vi "Write Count.vi"(8 "error in (no error)":errorcluster, 10 "Count":bool, 11 "TileTimer in":refnum<class "TileTimer.lvclass">) -> (0 "error out":errorcluster, 3 "TileTimer out":refnum<class "TileTimer.lvclass">)   [LabVIEW 2019, in "RT_Game.lvlib" / "TileTimer.lvclass"]
uses:
  TileTimer.lvclass
  TileTimer.lvclass/TileTimer.ctl
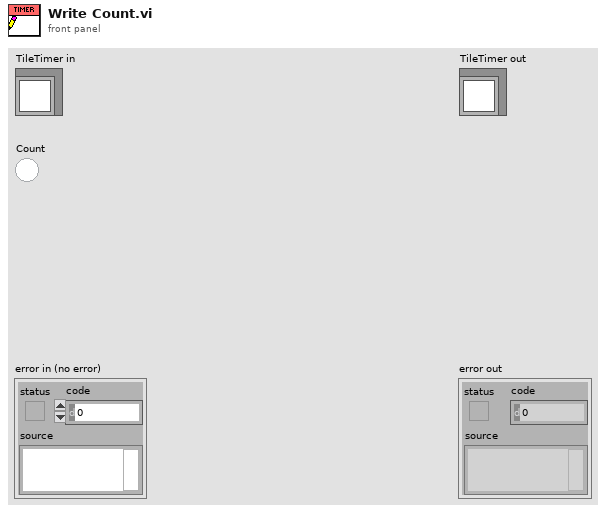
[diagram p1: front panel]
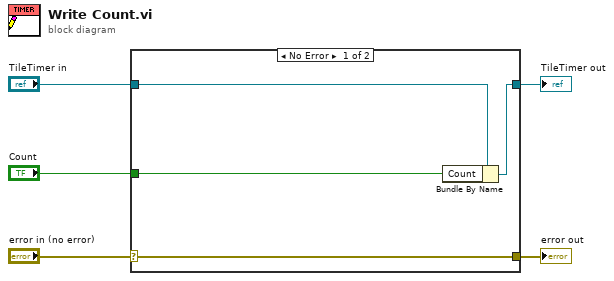
[diagram p0: block diagram]
diagram:
  n1 = case shown="No Error" "error in (no error)" {
    selector: "error in (no error)" -> [w9 w10]
    tunnel: [w9 w10] -> w4
    tunnel: [w7 w11] -> w2
    tunnel: "TileTimer in" -> [w8 w11]
    tunnel: "Count" -> [w6 _]
    frame No Error {
      n2 = Bundle By Name(cluster=w8, "Count"=w6) -> (w7:refnum<class "TileTimer.lvclass">)
    }
    frame Error {
    }
  }
  "error out" <- w4
  "TileTimer out" <- w2
